vi "Write Heap Save Format.vi"(8 "error in (no error)":errorcluster, 11 "Heap Save Format":T1=1 items=["Off", "XML", "Binary", "Verbose Tagged Text", "Binary2"]) -> (0 "error out":errorcluster)   [LabVIEW 2026, in "VILab.lvlib"]
uses:
  VILab.lvlib
  CTLs/Heap Save Format.ctl
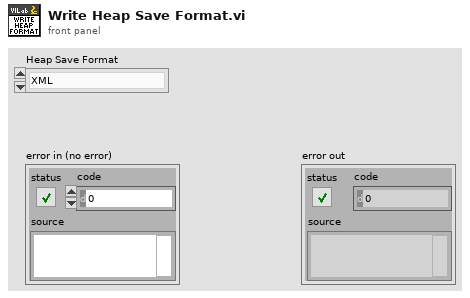
[diagram p1: front panel]
types:
  T1 = typedef "VILab.lvlib/Heap Save Format.ctl" = u16
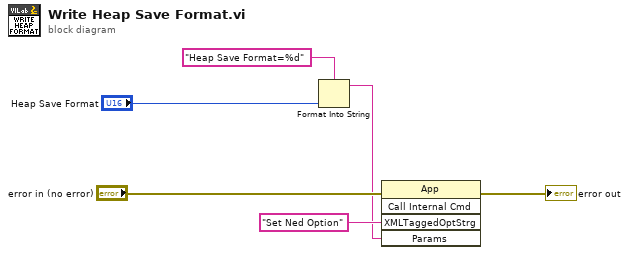
[diagram p0: block diagram]
diagram:
  n1 = Format Into String(format string="Heap Save Format=%d" ("initial string"), "Heap Save Format") -> (resulting string=w1:string)  [unwired: 2 in, 1 out]
  n2 = invoke class="App" method="Call Internal Cmd"(error in="error in (no error)", "XMLTaggedOptStrg"="Set Ned Option" ("Command Name"), "Params"=w1) -> (error out=→"error out":errorcluster)  [unwired: 2 in, 4 out]
